vi "UserDefined.Group.Message.Create.vi"(8 "error in (no error)":errorcluster, 10 "Message":T2 {"Signals"."Response"."Byte Order" items=["Little Endian", "Big Endian"]; "Signals"."Response"."Data Type" items=["Signed", "Unsigned", "IEEE Float"]; "Signals"."Cmd"."Byte Order" items=["Little Endian", "Big Endian"]; "Signals"."Cmd"."Data Type" items=["Signed", "Unsigned", "IEEE Float"]}, 11 "Section Ptr":T1 format="%.0x") -> (0 "error out":errorcluster, 3 "Parent Ref out":T1 format="%.0x")   [LabVIEW 2015, in "Diagnostics Addon System Explorer.lvlib"]
uses:
  Diagnostics Addon System Explorer.lvlib
  Types/UserDefined.Group.Message.Export.ctl
  Types/CmdResp.Export.ctl
  Shared/Types/Signal.ctl
  <vilib>/NI Veristand/Custom Device API/Custom Device Item Ref.ctl
  Types/FG.Action.ctl
  Shared/Types/Type.ctl
  <vilib>/NI Veristand/Custom Device API/Custom Device Channel.ctl
  <vilib>/NI Veristand/Custom Device API/Custom Device Channel Type.ctl
  <vilib>/NI Veristand/Custom Device API/NI VeriStand - Get Item Property.vi
  <vilib>/NI Veristand/Custom Device API/Get Item Property (U32).vi
  <vilib>/NI/NI VeriStand Advanced SysDef API/SysDef API/SysDef.Property.Set.vi
  <vilib>/NI/NI VeriStand Advanced SysDef API/_SubVIs/SysDef.Property.Set.U32.vi
  Shared/SubVIs/Constants.vi
  Shared/Diagnostics Addon Shared.lvlib
  <vilib>/NI VeriStand/Custom Device API/Custom Device API.lvlib
  <vilib>/NI/NI VeriStand Advanced SysDef API/SysDef API/Advanced System Definition.lvlib
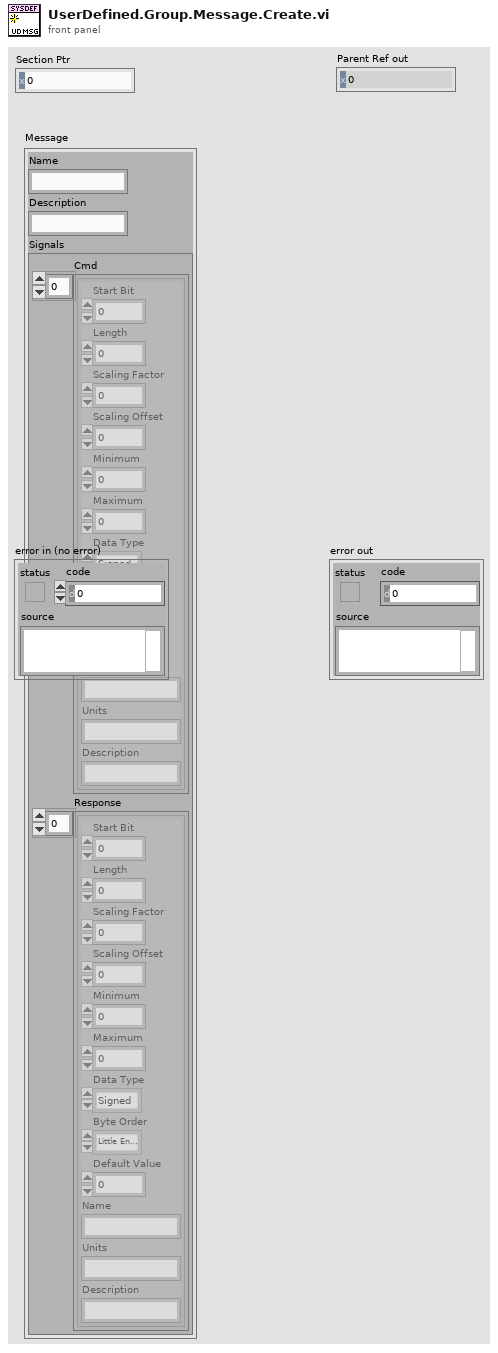
[diagram p1: front panel]
types:
  T1 = typedef "Custom Device API.lvlib/Custom Device Item Ref.ctl" = u64
  T2 = typedef "Diagnostics Addon System Explorer.lvlib/UserDefined.Group.Message.Export.ctl" = cluster{"Name":string, "Description":string, "Signals":T3}
  T3 = typedef "Diagnostics Addon System Explorer.lvlib/CmdResp.Export.ctl" = cluster{"Cmd":T4[], "Response":T4[]}
  T4 = typedef "Diagnostics Addon Shared.lvlib/Signal.ctl" = cluster{"Start Bit":u32, "Length":u32, "Scaling Factor":dbl, "Scaling Offset":dbl, "Minimum":dbl, "Maximum":dbl, "Data Type":u32, "Byte Order":u32, "Default Value":dbl, "Name":string, "Units":string, "Description":string}
  T5 = typedef "Custom Device API.lvlib/Custom Device Channel.ctl" = cluster{"Type":T6, "Units":string, "Default Value":dbl, "Faultable":bool, "Scalable":bool}
  T6 = typedef "Custom Device API.lvlib/Custom Device Channel Type.ctl" = enum16{"Input", "Output"}
  T7 = typedef "Diagnostics Addon Shared.lvlib/Type.ctl" = enum16{"DID", "CDID", "PID", "CPID", "Read Memory", "Write Memory", "DTC Control", "IO Cmd", "IO Resp", "Routine Start Cmd", "Routine Start Resp", "Routine Request Cmd", "Routine Request Resp", "Routine Stop Cmd", "Routine Stop Resp", "UserDefined Cmd", "UserDefined Rsp"}
  T8 = typedef "Diagnostics Addon System Explorer.lvlib/FG.Action.ctl" = enum16{"Get", "Set"}
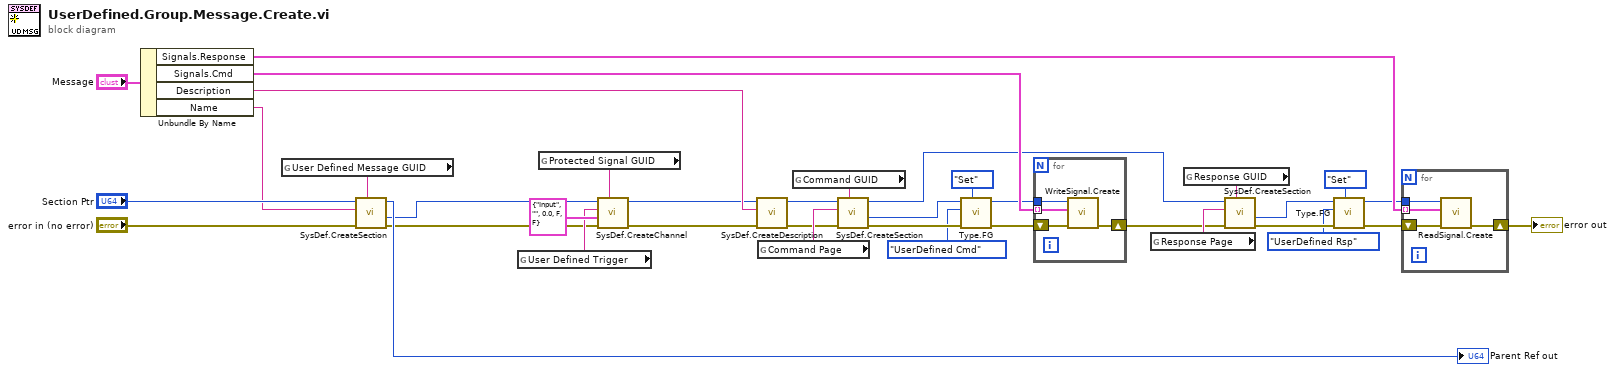
[diagram p0: block diagram]
diagram:
  n1 = Unbundle By Name("Message") -> ("Signals.Response"=w29:T4[], "Signals.Cmd"=w37:T4[], "Description"=w32:string, "Name"=w8:string)
  n2 = global read "Constants.vi" "User Defined Message GUID"() -> (w35:string)
  n3 = call <vilib>:"SysDef.CreateSection.vi"("GUID"=w35, "error in (no error)"="error in (no error)", "Name"=w8, "nodeID"="Section Ptr") -> ("error out"=w4:errorcluster, "New NodeID"=w2:u64, "nodeID out"=→"Parent Ref out":u64)  [unwired: 4 in, 1 out]
  n4 = global read "Constants.vi" "User Defined Trigger"() -> (w5:string)
  n5 = global read "Constants.vi" "Protected Signal GUID"() -> (w6:string)
  n6 = call <vilib>:"SysDef.CreateChannel.vi"("GUID"=w6, "error in (no error)"=w4, "Channel"=T5 {"Type"=enum."Input", "Units"="", "Default Value"=0.0, "Faultable"=FALSE, "Scalable"=FALSE}, "Name"=w5, "nodeID"=w2) -> ("error out"=w3:errorcluster, "nodeID out"=w1:u64)  [unwired: 3 in, 2 out]
  n7 = call <vilib>:"SysDef.CreateDescription.vi"("error in (no error)"=w3, "Description"=w32, "ID in"=w1) -> ("error out"=w23:errorcluster, "ID out"=w22:T1)  [unwired: 7 in]
  n8 = global read "Constants.vi" "Command Page"() -> (w28:string)
  n9 = global read "Constants.vi" "Command GUID"() -> (w27:string)
  n10 = call <vilib>:"SysDef.CreateSection.vi"("GUID"=w27, "error in (no error)"=w23, "Name"=w28, "nodeID"=w22) -> ("error out"=w18:errorcluster, "New NodeID"=w20:u64, "nodeID out"=w24:u64)  [unwired: 4 in, 1 out]
  n11 = call "Type.FG.vi"("Action"=FG.Action."Set", "error in (no error)"=w18, "Type"=Type."UserDefined Cmd", "Device Item Ref in"=w20) -> ("error out"=w17:errorcluster, "Device Item Ref out"=w19:T1)  [unwired: 5 in, 1 out]
  n12 = for {
    shift-right: [w38] -> w21
    shift-left: w17 -> [w41]
    tunnel: w37 -> [w40] mode=indexing
    tunnel: w19 -> [w39]
    n13 = call "WriteSignal.Create.vi"("error in (no error)"=w41, "Signal Parameters"=w40, "Section Ptr"=w39) -> ("error out"=w38:errorcluster)  [unwired: 7 in, 1 out]
  }
  n14 = global read "Constants.vi" "Response Page"() -> (w25:string)
  n15 = global read "Constants.vi" "Response GUID"() -> (w26:string)
  n16 = call <vilib>:"SysDef.CreateSection.vi"("GUID"=w26, "error in (no error)"=w21, "Name"=w25, "nodeID"=w24) -> ("error out"=w14:errorcluster, "New NodeID"=w12:u64)  [unwired: 4 in, 2 out]
  n17 = call "Type.FG.vi"("Action"=FG.Action."Set", "error in (no error)"=w14, "Type"=Type."UserDefined Rsp", "Device Item Ref in"=w12) -> ("error out"=w13:errorcluster, "Device Item Ref out"=w11:T1)  [unwired: 5 in, 1 out]
  n18 = for {
    shift-right: [w45] -> w30
    shift-left: w13 -> [w44]
    tunnel: w29 -> [w43] mode=indexing
    tunnel: w11 -> [w42]
    n19 = call "ReadSignal.Create.vi"("error in (no error)"=w44, "Signal Parameters"=w43, "Section Ptr"=w42) -> ("error out"=w45:errorcluster)  [unwired: 7 in, 1 out]
  }
  "error out" <- w30
